vi "Fifo_measurement_example modified.vi"(3 "Required No of photons":u32=10000, 4 "append to file? (new file:F)":bool, 5 "file path (dialog if empty)":path) -> (0 "SPC error":T2={"Error code"=0, "Message"="No errors"})   [LabVIEW 2012]
uses:
  spcm_functions_lv10.llb/error.ctl
  spcm_functions_lv10.llb/SPC_mod_info.ctl
  spcm_functions_lv10.llb/Global_SPCM_vars.vi
  Global FIFO variabls.vi
panel:
  out "Fifo type":i16(ring)=5 items=["48 bits SPC-6x0", "32 bits SPC-6x0", "32 bits SPC-130", "32 bits SPC-830", "32 bits SPC-140", "32 bits SPC-150", "32 bits DPC-230", "32 bits FIFO_IMAGE"]
  out "?":string="SPC-7x0 module cannot work in FIFO mode"
  out "MT clock [ns]":dbl
  out "Rout Channel":u16[](array[numeric]) format="%0.0f"
  out "Micro Time":u16[](array[numeric]) format="%04.0f"
  out "Macro Time Low":u32[](array[numeric]) format="%08x"
  out "No of extracted photons":u32
  out "Frames":u16[][](array[numeric]) format="%04x"
  out "Data Buffer":u16[](array[numeric]) format="%04x"
  in  "Frames per call":u32=4096 min=1 max=1000000
  out "Words per frame":u32
  out "No of read frames":u32
  out "FIFO Overflow":bool
  in  "Stop Button":bool
  in  "Frame size for SPC-6x0":sgl(ring)=3.0 items=["32 bits"=3, "48 bits"=2]
  out "?":string="SPC-7x0 module cannot work in FIFO mode"
  out "SPC module info":T1={"module type"=130, "bus number"=3, "slot number"=10, "in use"=1, "init status"=0, "base I/O addr"=0} {"bus number" min=0 max=255 step=1; "base I/O addr" format="%.0x"; "init status" min=-10 max=0 step=1; "in use" min=-1 max=1 step=1; "slot number" min=0 max=255 step=1; "module type" min=-32767 step=1}
  in  "Active module":u16(ring) items=["Module 0", "Module 1", "Module 2", "Module 3", "Module 4", "Module 5", "Module 6", "Module 7"]
  out "Modules in use":T3={"M0"=TRUE, "M1"=FALSE, "M2"=FALSE, "M3"=FALSE, "M4"=FALSE, "M5"=FALSE, "M6"=FALSE, "M7"=FALSE}
  # "FIFO Measurement Example for SPC modules\nB&H, 2008"
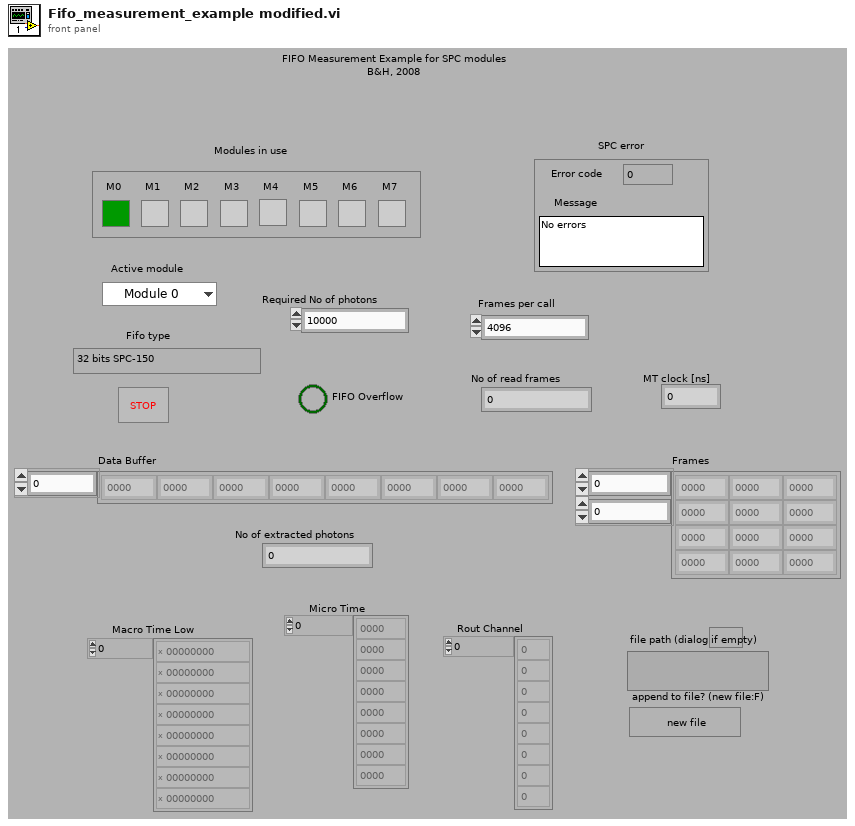
[diagram p1: front panel]
types:
  T1 = typedef "SPC_mod_info.ctl" = cluster{"module type":i16, "bus number":i16, "slot number":i16, "in use":i16, "init status":i16, "base I/O addr":u16}
  T2 = typedef "error.ctl" = cluster{"Error code":i16, "Message":string}
  T3 = cluster{"M0":bool, "M1":bool, "M2":bool, "M3":bool, "M4":bool, "M5":bool, "M6":bool, "M7":bool}
  T4 = typedef "SPC_PhotStreamInfo.ctl" = cluster{"Fifo type":i16, "Stream type":i16, "Macro time clock [0.1ns]":i32, "Rout channels":i16, "What to read":i16, "No of files in stream":i16, "No of ready files":i16, "Stream base name":string, "1st file number":i16, "Current file number":i16, "Current file name":string, "Stream size":u32, "Current offset in stream":u32, "Offset in current file":u32, "No of fifo overruns":i32, "No of invalid photons":i32, "No of read photons":i32, "No of read markers 0 (pixel )":i32, "No of read markers 1 (line )":i32, "No of read markers 2 (frame )":i32, "Start offset of 1st photon ( only DPC-230)":i32, "No of read markers 3":i32}
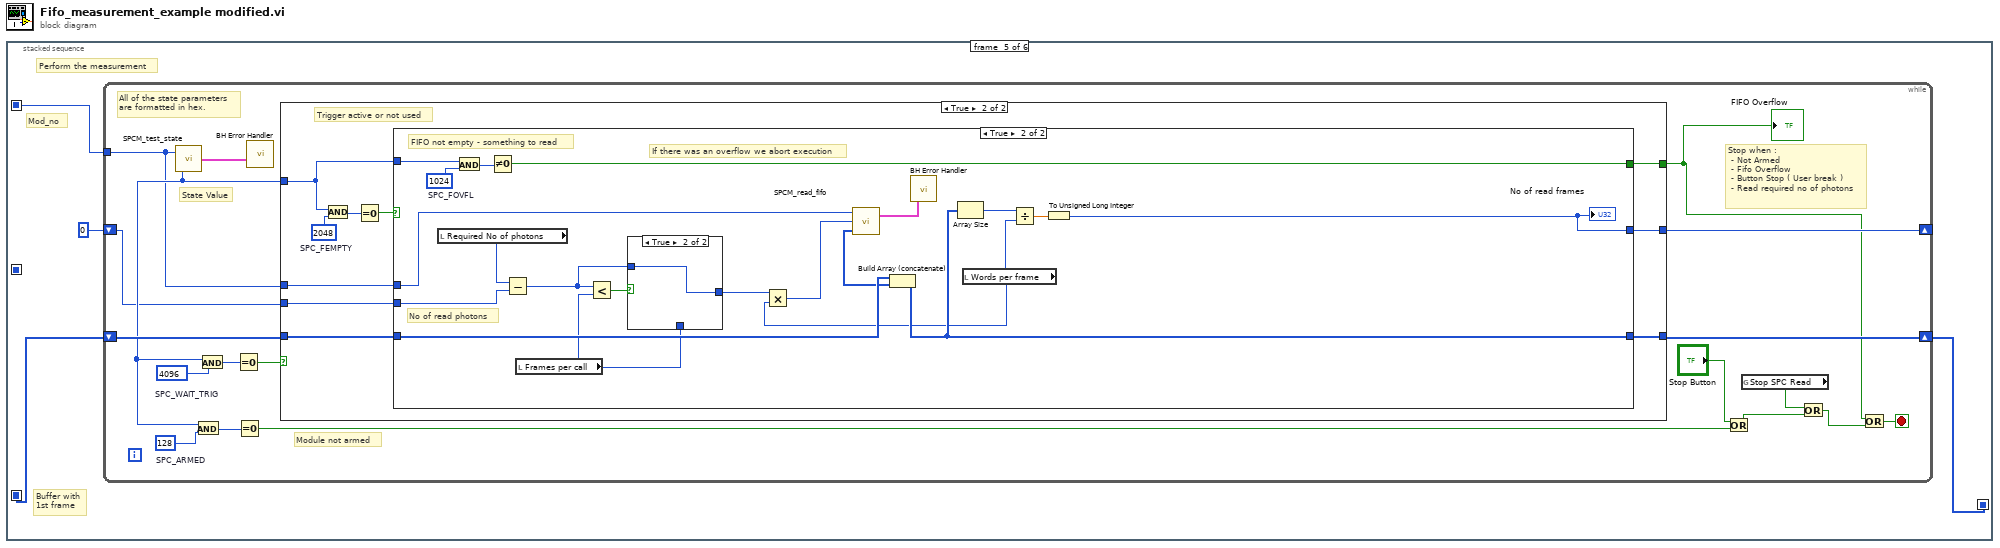
[diagram p0: block diagram]
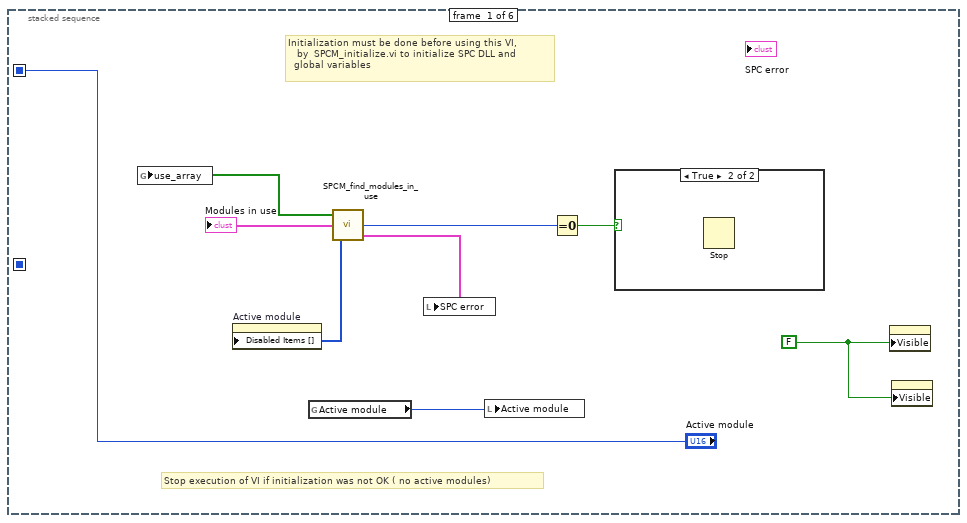
[diagram p2: hidden frame]
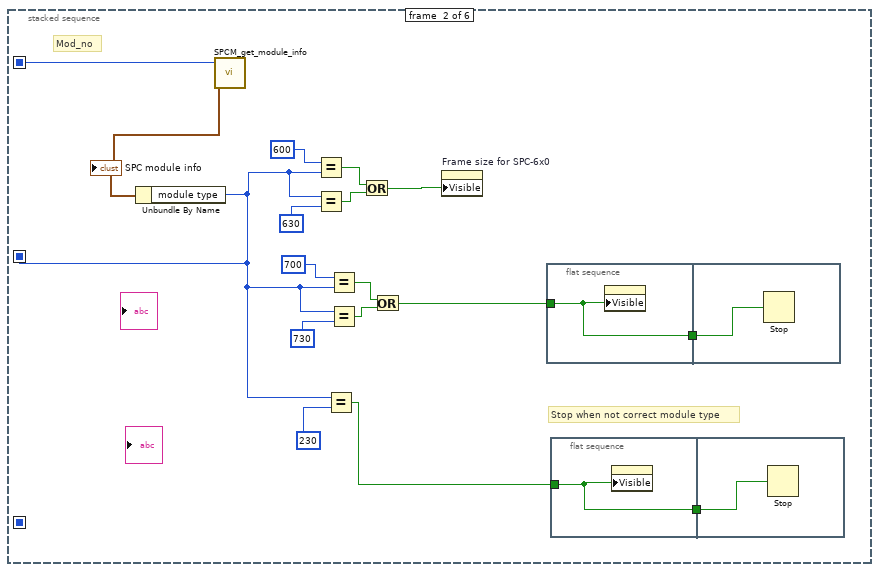
[diagram p4: hidden frame]
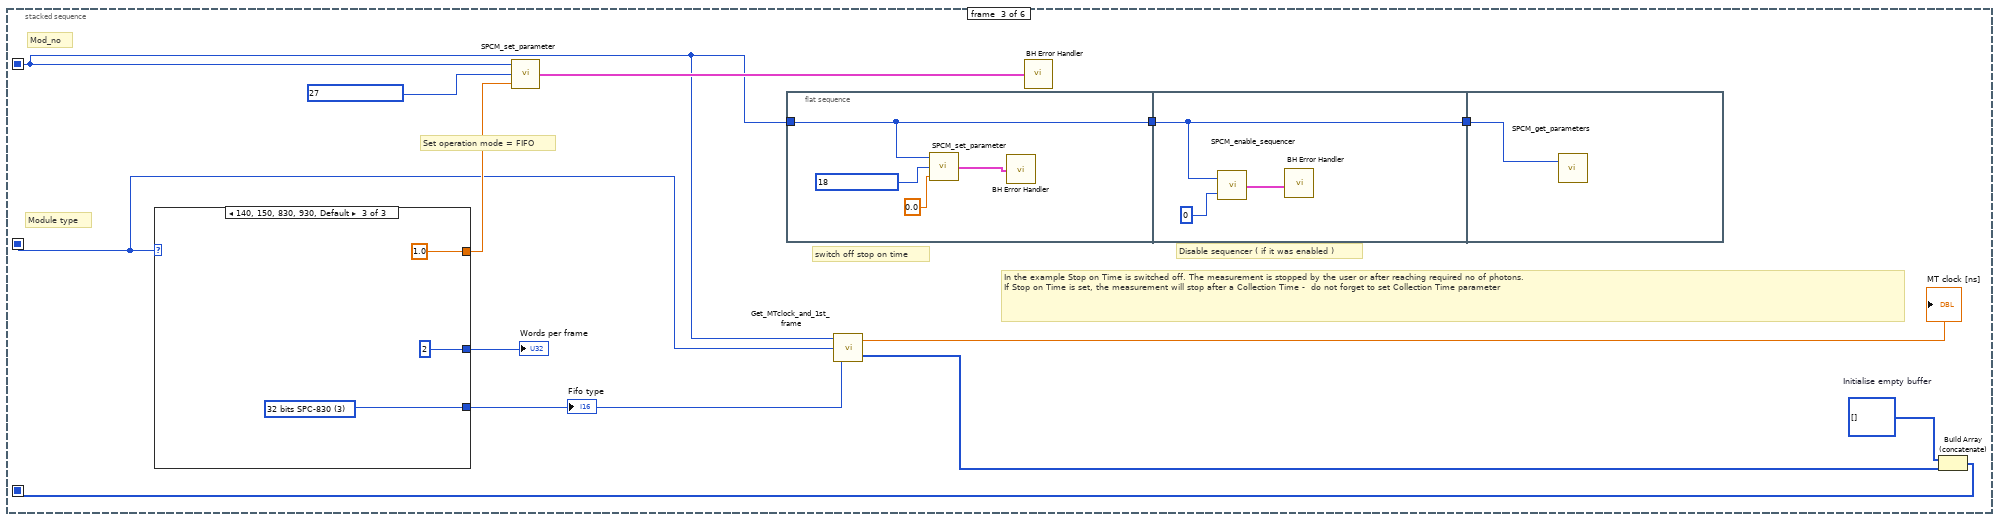
[diagram p5: hidden frame]
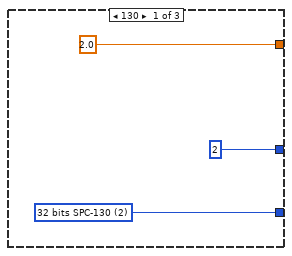
[diagram p6: hidden frame]
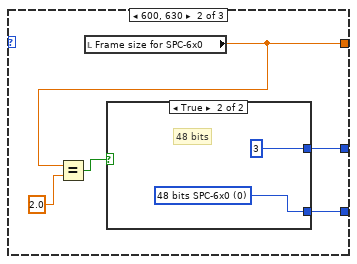
[diagram p7: hidden frame]
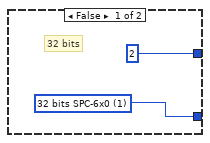
[diagram p8: hidden frame]
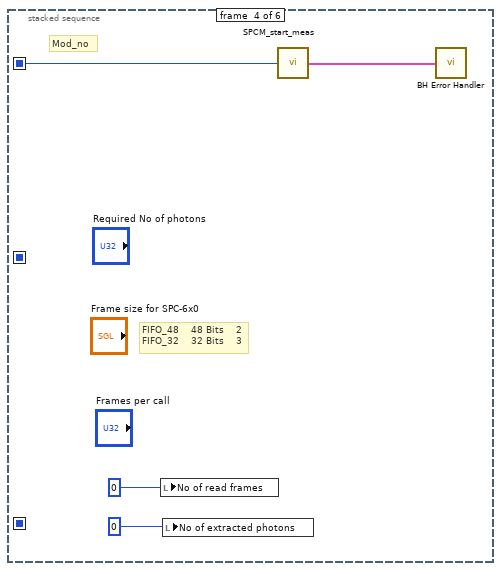
[diagram p9: hidden frame]
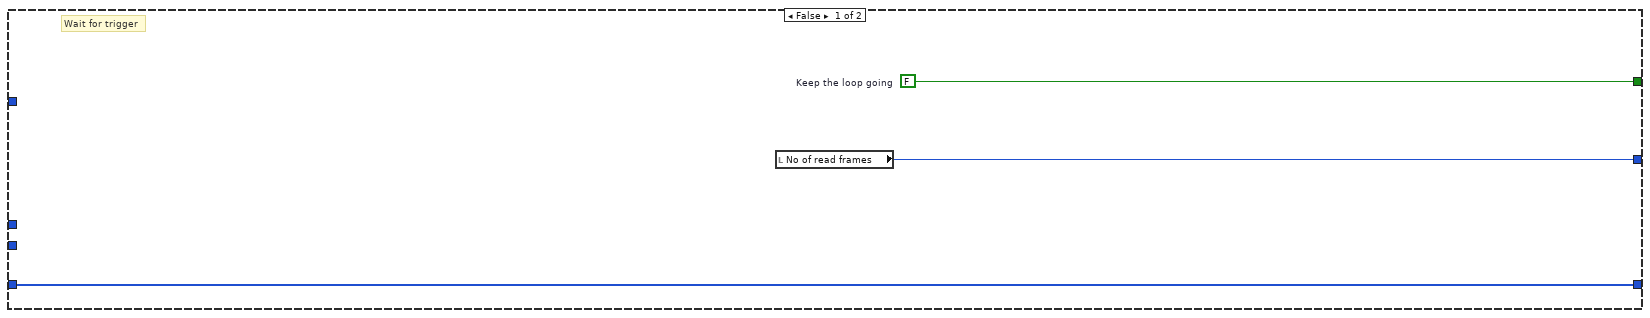
[diagram p10: hidden frame]
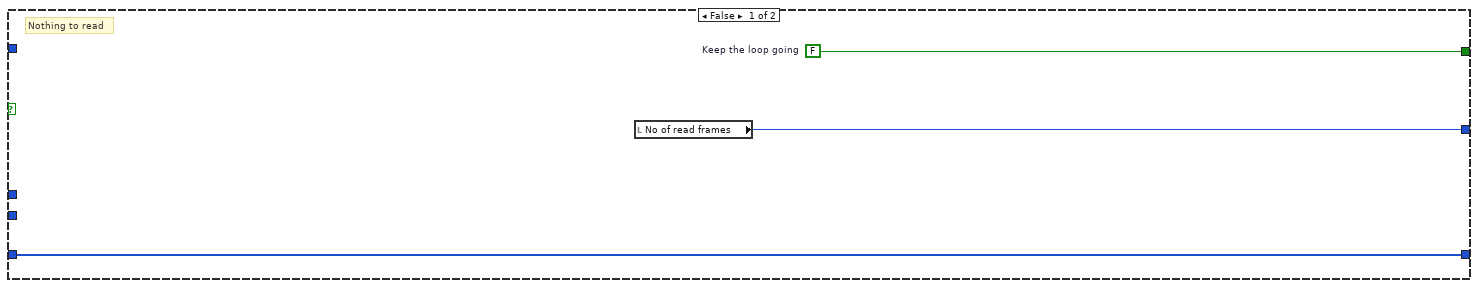
[diagram p11: hidden frame]
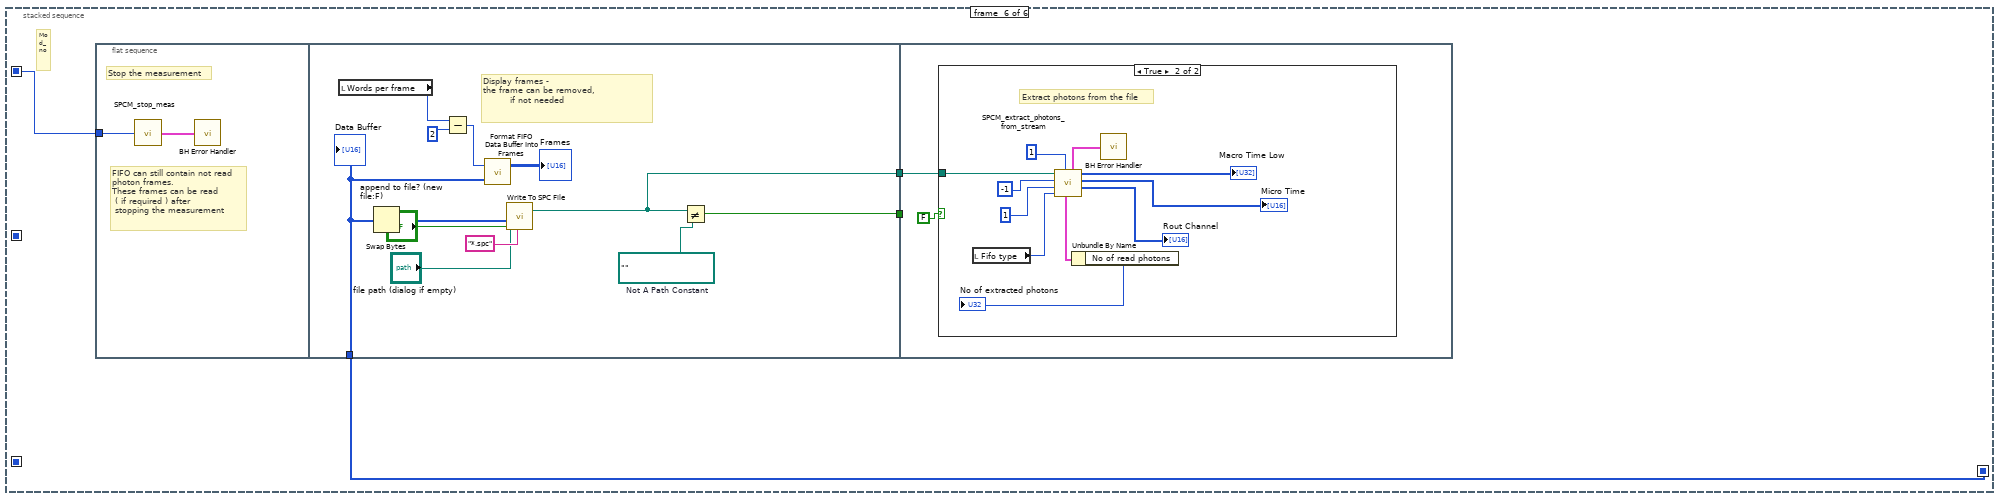
[diagram p13: hidden frame]
diagram:
  n1 = stacked-sequence {
    seq-local: ["Active module" _ _ _ _ _] -> [_ w17 w38 w70 w74 w135]
    seq-local: [_ w11 _ _ _ _] -> [_ _ w37 _ _ _]
    seq-local: [_ _ _ _ w72 _] -> [_ _ _ _ _ w134]
    seq-local: [_ _ w39 _ _ _] -> [_ _ _ _ w71 _]
    frame #0 {
      w1 = FALSE ("Visible")
      # "Stop execution of VI if initialization was not OK ( no active modules)"
      # "Initialization must be done before using this VI, \n   by  SPCM_initialize.vi to initialize SPC DLL and \n  global variables"
      n2 = global read "Global_SPCM_vars.vi" "Active module"() -> (w4:i16)
      n3 = call "SPCM_find_modules_in_use.vi"() -> ("SPC error"=w8:T2, "Number of used modules"=w6:i16, "Disabled Items"=w5:i32[], "Use LEDs"=→"Modules in use":T3, "use_array"=w3:bool[])  [unwired: 1 out]
      n4 = global write "Global_SPCM_vars.vi" "use_array"(w3) -> ()
      n5 = property on="Active module" class="Ring (strict)"("Disabled Items []"=w5) -> ()  [unwired: 2 in, 2 out]
      n6 = local write "SPC error"(w8) -> ()
      n7 = local write "Active module"(w4) -> ()
      n8 = Equal To 0?(x=w6) -> (x = 0?=w7:bool)
      n9 = case shown="True" w7 {
        frame False {
        }
        frame True {
          n10 = Stop() -> ()  [unwired: 1 in]
        }
      }
      n11 = property class="Str"("Visible"=w1) -> ()  [unwired: 2 in, 2 out]
      n12 = property class="Str"("Visible"=w1) -> ()  [unwired: 2 in, 2 out]
    }
    frame #1 {
      # "Mod_no"
      # "Stop when not correct module type"
      n13 = call "SPCM_get_module_info.vi"("Module no"=w17) -> ("SPC module info"=w26:T1)  [unwired: 1 out]
      "SPC module info" <- w26
      n14 = Unbundle By Name(w26) -> ("module type"=w11:i16)
      n15 = Equal?(x=i16 600, y=w11) -> (x = y?=w23:bool)
      n16 = Equal?(x=w11, y=i16 630 ("x")) -> (x = y?=w22:bool)
      n17 = Equal?(x=w11, y=230) -> (x = y?=w10:bool)
      n18 = Equal?(x=i16 700, y=w11) -> (x = y?=w19:bool)
      n19 = Equal?(x=w11, y=i16 730 ("x")) -> (x = y?=w18:bool)
      n20 = Or(x=w23, y=w22) -> (x .or. y?=w16:bool)
      n21 = Or(x=w19, y=w18) -> (x .or. y?=w15:bool)
      n22 = property on="Frame size for SPC-6x0" class="Ring (strict)"("Visible"=w16) -> ()  [unwired: 2 in, 2 out]
      n23 = flat-sequence {
        tunnel: w15 -> [w29]
        tunnel: [w29] -> w14
        tunnel: w14 -> [w30]
        frame #0 {
          n24 = property class="Str"("Visible"=w29) -> ()  [unwired: 2 in, 2 out]
        }
        frame #1 {
          n25 = Stop(stop? (T)=w30) -> ()
        }
      }
      n26 = flat-sequence {
        tunnel: [w27] -> w13
        tunnel: w10 -> [w27]
        tunnel: w13 -> [w28]
        frame #0 {
          n27 = property class="Str"("Visible"=w27) -> ()  [unwired: 2 in, 2 out]
        }
        frame #1 {
          n28 = Stop(stop? (T)=w28) -> ()
        }
      }
    }
    frame #2 {
      w40 = u16[] []  # Initialise empty buffer
      # "In the example Stop on Time is switched off. The measurement is stopped by the user or after reaching required no of photons.\nIf Stop on Time is set, the measurement will stop after a Collection Time -  do not forget to set Collection Time parameter"
      # "switch off stop on time"
      # "Disable sequencer ( if it was enabled )"
      # "Set operation mode = FIFO"
      # "Module type"
      # "Mod_no"
      n29 = case shown="140, 150, 830, 930, Default" w37 {
        tunnel: [sgl 2.0 w58 sgl 1.0] -> w43
        tunnel: [2 w56 2] -> w42
        tunnel: [w52 w55 w64] -> w34
        frame 130 {
          w52 = i16 2 items=["48 bits SPC-6x0", "32 bits SPC-6x0", "32 bits SPC-130", "32 bits SPC-830", "32 bits SPC-140", "32 bits SPC-150", "32 bits DPC-230", "32 bits FIFO_IMAGE"] ("Fifo type")
        }
        frame 600, 630 {
          n30 = local read "Frame size for SPC-6x0"() -> (w58:sgl)
          n31 = Equal?(x=w58, y=sgl 2.0) -> (x = y?=w59:bool)
          n32 = case shown="True" w59 {
            tunnel: [2 3] -> w56
            tunnel: [w60 w62] -> w55
            frame False {
              w60 = i16 1 items=["48 bits SPC-6x0", "32 bits SPC-6x0", "32 bits SPC-130", "32 bits SPC-830", "32 bits SPC-140", "32 bits SPC-150", "32 bits DPC-230", "32 bits FIFO_IMAGE"] ("Fifo type")
              # "32 bits"
            }
            frame True {
              w62 = i16 0 items=["48 bits SPC-6x0", "32 bits SPC-6x0", "32 bits SPC-130", "32 bits SPC-830", "32 bits SPC-140", "32 bits SPC-150", "32 bits DPC-230", "32 bits FIFO_IMAGE"] ("Fifo type")
              # "48 bits"
            }
          }
        }
        frame 140, 150, 830, 930, Default {
          w64 = i16 3 items=["48 bits SPC-6x0", "32 bits SPC-6x0", "32 bits SPC-130", "32 bits SPC-830", "32 bits SPC-140", "32 bits SPC-150", "32 bits DPC-230", "32 bits FIFO_IMAGE"] ("Fifo type")
        }
      }
      "Words per frame" <- w42
      "Fifo type" <- w34
      n33 = call "SPCM_set_parameter.vi"("Parameter Value"=w43, "SPC parameter ID"=u16 27, "Module no"=w38) -> ("SPC error"=w41:cluster{"Error code":i16, "Message":string})
      n34 = flat-sequence {
        tunnel: w38 -> [w46]
        tunnel: [w46] -> w33
        tunnel: w33 -> [w48]
        tunnel: [w48] -> w31
        tunnel: w31 -> [w51]
        frame #0 {
          n35 = call "SPCM_set_parameter.vi"("Parameter Value"=sgl 0.0, "SPC parameter ID"=u16 18, "Module no"=w46) -> ("SPC error"=w47:cluster{"Error code":i16, "Message":string})
          n36 = call "BH Error Handler.vi"("B&H Error Code In"=w47) -> ()  [unwired: 1 in]
        }
        frame #1 {
          n37 = call "SPCM_enable_sequencer.vi"("Enable"=i16 0, "Module no"=w48) -> ("SPC error"=w49:cluster{"Error code":i16, "Message":string})
          n38 = call "BH Error Handler.vi"("B&H Error Code In"=w49) -> ()  [unwired: 1 in]
        }
        frame #2 {
          n39 = call "SPCM_get_parameters.vi"("Module no"=w51) -> ()  [unwired: 2 out]
        }
      }
      n40 = call "Get_MTclock_and_1st_frame.vi"("Fifo type"=w34, "module type"=w37, "module no"=w38) -> ("1st Frame"=w36:u16[], "MT clock [ns]"=→"MT clock [ns]":dbl)
      n41 = call "BH Error Handler.vi"("B&H Error Code In"=w41) -> ()  [unwired: 1 in]
      n42 = Build Array (concatenate)(w40, w36) -> (w39:u16[])
    }
    frame #3 {
      # "Mod_no"
      # "FIFO_48    48 Bits    2\nFIFO_32    32 Bits    3"
      n43 = local write "No of read frames"(0 ("No of read photons")) -> ()
      n44 = local write "No of extracted photons"(u32 0 ("No of extracted photons")) -> ()
      n45 = call "SPCM_start_meas.vi"("Module no"=w70) -> ("SPC error"=w69:cluster{"Error code":i16, "Message":string})
      n46 = call "BH Error Handler.vi"("B&H Error Code In"=w69) -> ()  [unwired: 1 in]
    }
    frame #4 {
      # "Buffer with\n1st frame"
      # "Mod_no"
      # "Perform the measurement"
      n47 = while {
        shift-right: [w79] -> w72
        shift-left: w71 -> [w93]
        tunnel: w74 -> [w83]
        shift-right: [w80] -> _
        shift-left: 0 ("No of read photons") -> [w81]
        stop <- w91 stop-if-true
        w89 = i16 128  # SPC_ARMED
        w86 = i16 4096  # SPC_WAIT_TRIG
        # "Module not armed"
        # "Stop when :\n - Not Armed\n - Fifo Overflow\n - Button Stop ( User break )\n - Read required no of photons"
        # "State Value"
        # "All of the state parameters \nare formatted in hex."
        n48 = call "SPCM_test_state.vi"("Module no"=w83) -> ("SPC error"=w90:cluster{"Error code":i16, "Message":string}, "state value"=w84:i16)
        n49 = And(x=w84, y=w89) -> (x .and. y?=w88:i16)
        n50 = And(x=w84, y=w86) -> (x .and. y?=w85:i16)
        n51 = Equal To 0?(x=w85) -> (x = 0?=w92:bool)
        n52 = Equal To 0?(x=w88) -> (x = 0?=w87:bool)
        n53 = call "BH Error Handler.vi"("B&H Error Code In"=w90) -> ()  [unwired: 1 in]
        n54 = case shown="True" w92 {
          tunnel: w84 -> [_ w104]
          tunnel: [w96 w101] -> w75
          tunnel: [w95 w100] -> w79
          tunnel: w93 -> [w95 w105]
          tunnel: w83 -> [_ w99]
          tunnel: [w94 w98] -> w80
          tunnel: w81 -> [_ w97]
          frame False {
            w96 = FALSE  # Keep the loop going
            # "Wait for trigger"
            n55 = local read "No of read frames"() -> (w94:u32)
          }
          frame True {
            w103 = i16 2048  # SPC_FEMPTY
            # "Trigger active or not used"
            n56 = And(x=w104, y=w103) -> (x .and. y?=w102:i16)
            n57 = Equal To 0?(x=w102) -> (x = 0?=w106:bool)
            n58 = case shown="True" w106 {
              tunnel: w104 -> [_ w128]
              tunnel: [w109 w127] -> w101
              tunnel: [w108 w124] -> w100
              tunnel: w105 -> [w108 w126]
              tunnel: w99 -> [_ w121]
              tunnel: [w107 w110] -> w98
              tunnel: w97 -> [_ w113]
              frame False {
                w109 = FALSE  # Keep the loop going
                # "Nothing to read"
                n59 = local read "No of read frames"() -> (w107:u32)
              }
              frame True {
                w123 = i16 1024  # SPC_FOVFL
                # "No of read photons"
                # "If there was an overflow we abort execution"
                # "FIFO not empty - something to read"
                n60 = local read "Required No of photons"() -> (w114:u32)
                n61 = And(x=w128, y=w123) -> (x .and. y?=w122:i16)
                n62 = Not Equal To 0?(x=w122) -> (x != 0?=w127:bool)
                n63 = Subtract(x=w114, y=w113) -> (x-y=w117:u32)
                n64 = local read "Frames per call"() -> (w118:u32)
                n65 = Less?(x=w117, y=w118) -> (x < y?=w119:bool)
                n66 = case shown="True" w119 {
                  tunnel: [w130 w131] -> w116
                  tunnel: w118 -> [w130 _]
                  tunnel: w117 -> [_ w131]
                  frame False {
                  }
                  frame True {
                  }
                }
                n67 = local read "Words per frame"() -> (w112:u32)
                n68 = Multiply(x=w116, y=w112) -> (x*y=w115:u32)
                n69 = call "SPCM_read_fifo.vi"("Input Count"=w115, "Module no"=w121) -> ("SPC error"=w129:cluster{"Error code":i16, "Message":string}, "Data Buffer"=w125:u16[])  [unwired: 1 out]
                n70 = Build Array (concatenate) "Build Array"(w126, w125) -> (w124:u16[])
                n71 = call "BH Error Handler.vi"("B&H Error Code In"=w129) -> ()  [unwired: 1 in]
                n72 = Array Size(array=w124) -> (size(s)=w120:i32)
                n73 = Divide(x=w120, y=w112) -> (x/y=w111:dbl)
                n74 = To Unsigned Long Integer(number=w111) -> (unsigned 32bit integer=w110:u32)
                "No of read frames" <- w110
              }
            }
          }
        }
        "FIFO Overflow" <- w75
        n75 = Or(x="Stop Button", y=w87) -> (x .or. y?=w78:bool)
        n76 = global read "Global FIFO variabls.vi" "Stop SPC Read"() -> (w76:bool)
        n77 = Or(x=w76, y=w78) -> (x .or. y?=w77:bool)
        n78 = Or(x=w75, y=w77) -> (x .or. y?=w91:bool)
      }
    }
    frame #5 {
      # "Mod_no"
      n79 = flat-sequence {
        tunnel: w135 -> [w136]
        tunnel: w134 -> [w147]
        tunnel: [w142] -> w133
        tunnel: [w140] -> w132
        tunnel: w132 -> [w151]
        tunnel: w133 -> [_]
        frame #0 {
          # "FIFO can still contain not read\nphoton frames.\nThese frames can be read \n ( if required ) after\n stopping the measurement"
          # "Stop the measurement"
          n80 = call "SPCM_stop_meas.vi"("Module no"=w136) -> ("SPC error"=w137:cluster{"Error code":i16, "Message":string})
          n81 = call "BH Error Handler.vi"("B&H Error Code In"=w137) -> ()  [unwired: 1 in]
        }
        frame #1 {
          w141 = path ""  # Not A Path Constant
          # "Display frames -\nthe frame can be removed,\n         if not needed"
          n82 = local read "Words per frame"() -> (w143:u32)
          n83 = Swap Bytes(anything=w147) -> (byte swapped=w149:u16[])
          n84 = Subtract(x=w143, y=2) -> (x-y=w145:u32)
          n85 = call "Format FIFO Data Buffer Into Frames.vi"("Input data buffer"=w147, "Frame size"=w145) -> ("Frames H"=→"Frames":u16[][])  [unwired: 1 out]
          n86 = call "Write To SPC File.vi"("pattern"="*.spc", "append to file? (new file:F)"="append to file? (new file:F)", "1D array"=w149, "file path (dialog if empty)"="file path (dialog if empty)") -> ("new file path (Not A Path if cancelled)"=w140:path)  [unwired: 3 in]
          n87 = Not Equal?(x=w140, y=w141) -> (x != y?=w142:bool)
          "Data Buffer" <- w147
        }
        frame #2 {
          n88 = case shown="True" FALSE {
            tunnel: w151 -> [_ w161]
            frame False {
              # "User does not select any file path, operation cancelled"
            }
            frame True {
              # "Extract photons from the file"
              n89 = local read "Fifo type"() -> (w158:i16)
              n90 = call "SPCM_extract_photons_from_stream.vi"("Ignore invalid photons"=i16 1, "Fifo type"=w158, "BH SPC file type"=u32 1, "No of files to use"=i16 -1, "file path (dialog if empty)"=w161) -> ("Rout Channel"=→"Rout Channel":u16[], "Micro Time"=→"Micro Time":u16[], "Macro Time Low"=→"Macro Time Low":u32[], "SPC error"=w162:cluster{"Error code":i16, "Message":string}, "SPC_PhotStreamInfo"=w156:T4)  [unwired: 2 out]
              n91 = Unbundle By Name(w156) -> ("No of read photons"=→"No of extracted photons":i32)
              n92 = call "BH Error Handler.vi"("B&H Error Code In"=w162) -> ()  [unwired: 1 in]
            }
          }
        }
      }
    }
  }
